vi "Get Tamer Picture.vi"() -> (0 "Tamer":picture)   [LabVIEW 2026, in "TALOS.lvlib"]
uses:
  TALOS.lvlib
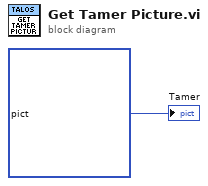
[diagram p0: block diagram]
diagram:
  "Tamer" <- picture bytes[51230] ("Tamer")
